vi "LMove.vi"(0 "reference in":refnum<class "Redis.lvclass">, 5 "Source":string, 7 "Destination":string, 9 "WhereFrom":T1, 11 "Error In":errorcluster, 12 "WhereTo":T1) -> (4 "reference out":refnum<class "Redis.lvclass">, 8 "Return":string, 15 "Error Out":errorcluster)   [LabVIEW 2020, in "Redis.lvclass"]
doc: "<b>LMOVE</b>\n\nAtomically returns and removes the first/last element (head/tail depending on the wherefrom argument) of the list stored at source, and pushes the element at the first/last element (head/tail depending on the whereto argument) of the list stored at destination.\n\nFor example: consider source holding the list a,b,c, and destination holding the list x,y,z. Executing LMOVE source destination RIGHT LEFT results in source holding a,b and destination holding c,x,y,z.\n\nIf source does not exist, the value nil is returned and no operation is performed. If source and destination are the same, the operation is equivalent to removing the first/last element from the list and pushing it as first/last element of the list, so it can be considered as a list rotation command (or a no-op if wherefrom is the same as whereto).\n\nThis command comes in place of the now deprecated <b>RPOPLPUSH</b>. Doing LMOVE RIGHT LEFT is equivalent."
uses:
  Redis.lvclass
  Redis.lvclass/Redis.ctl
  SideEnum.ctl
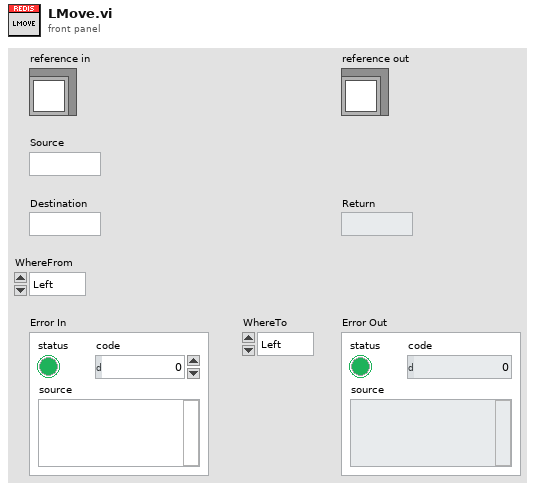
[diagram p1: front panel]
types:
  T1 = typedef "Redis.lvclass/SideEnum.ctl" = enum16{"Left", "Right"}
  T2 = typedef "Redis.lvclass/RedisDataType.ctl" = cluster{"Reply Type":T3, "Integer":i64, "String":string, "Multibulk":variant[], "StringData":string[]}
  T3 = typedef "Redis.lvclass/ReplyDataTypeEnum.ctl" = enum16{"None", "Error", "Status", "Nil", "Integer", "String", "Multibulk"}
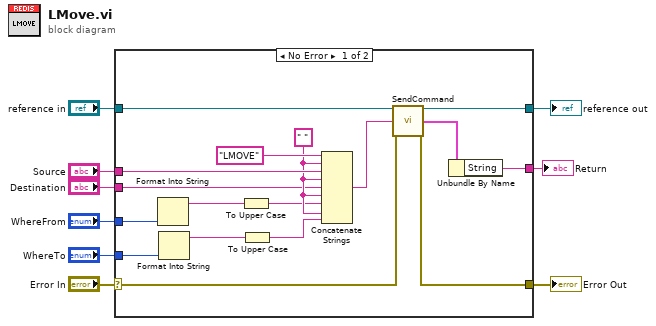
[diagram p0: block diagram]
diagram:
  n1 = case shown="No Error" "Error In" {
    selector: "Error In" -> [w24 w28]
    tunnel: [w23 w28] -> w8
    tunnel: [w26 w27] -> w6
    tunnel: "reference in" -> [w25 w27]
    tunnel: [w15 _] -> w3
    tunnel: "Source" -> [w20 _]
    tunnel: "WhereFrom" -> [w18 _]
    tunnel: "Destination" -> [w14 _]
    tunnel: "WhereTo" -> [w11 _]
    frame No Error {
      w16 = " "
      n2 = Format Into String(w18) -> (resulting string=w17:string)  [unwired: 3 in, 1 out]
      n3 = Format Into String(w11) -> (resulting string=w12:string)  [unwired: 3 in, 1 out]
      n4 = To Upper Case(1:w17) -> (0:w13:string)
      n5 = To Upper Case(1:w12) -> (0:w10:string)
      n6 = Concatenate Strings("LMOVE", w16, w20, w16, w14, w16, w13, w16, w10) -> (w19:string)
      n7 = call "SendCommand.vi"("reference in"=w25, "Command"=w19, "Error In"=w24) -> ("reference out"=w26:refnum<class "Redis.lvclass">, "Data"=w22:T2, "Error Out"=w23:errorcluster)  [unwired: 10 in]
      n8 = Unbundle By Name(w22) -> ("String"=w15:string)
    }
    frame Error {
    }
  }
  "Error Out" <- w8
  "reference out" <- w6
  "Return" <- w3
